vi "ws_users logout user.vi"(6 "Current User":T2, 7 "httpRequestID":u32, 8 "error in (no error)":errorcluster, 10 "Username to Logout (\"\")":string, 11 "Connection Refnum":T1) -> (0 "error out":errorcluster, 3 "Connection Refnum":T1)   [LabVIEW 2011]
uses:
  server/database/Users/User Record.ctl
  SI.LIB/ODBC/SQL Controls/Connection Refnum.ctl
  <vilib>/wsapi/NI_WebServices.lvlib
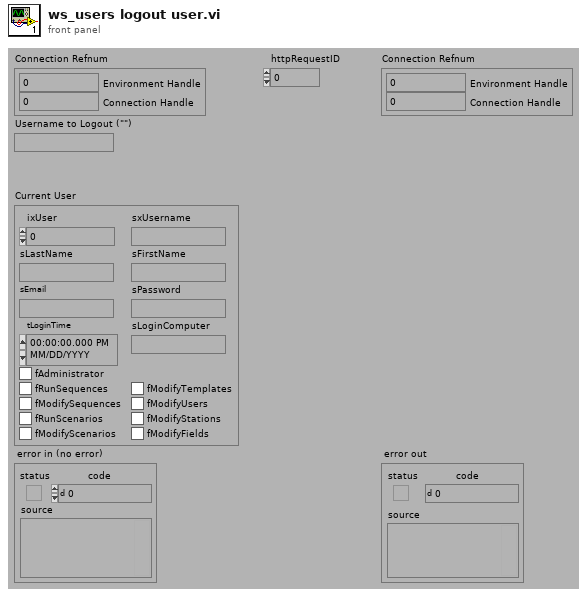
[diagram p1: front panel]
types:
  T1 = typedef "Connection Refnum.ctl" = cluster{"Environment Handle":i32, "Connection Handle":i32}
  T2 = typedef "User Record.ctl" = cluster{"ixUser":i32, "sxUsername":string, "sLastName":string, "sFirstName":string, "sEmail":string, "sPassword":string, "tLoginTime":timestamp, "sLoginComputer":string, "fAdministrator":bool, "fRunSequences":bool, "fModifySequences":bool, "fRunScenarios":bool, "fModifyScenarios":bool, "fModifyTemplates":bool, "fModifyUsers":bool, "fModifyStations":bool, "fModifyFields":bool}
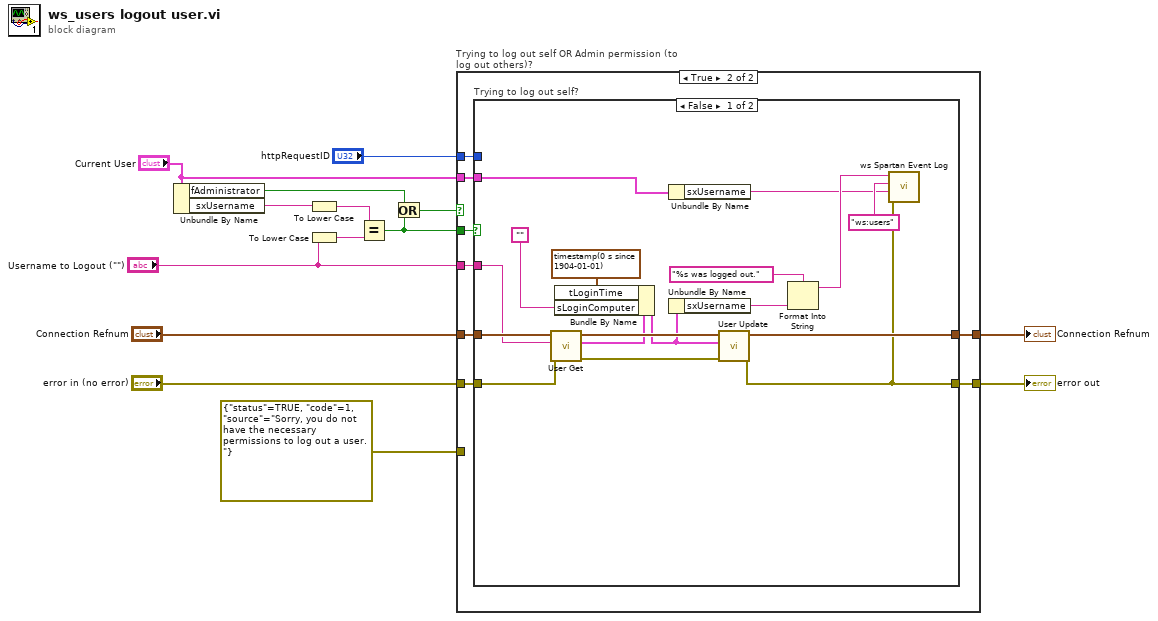
[diagram p0: block diagram]
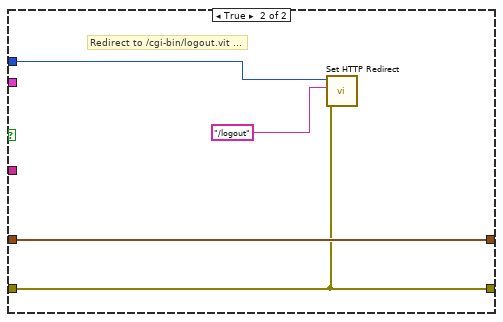
[diagram p3: hidden frame]
diagram:
  n1 = Unbundle By Name("Current User") -> ("fAdministrator"=w6:bool, "sxUsername"=w8:string)
  n2 = To Lower Case(string=w8) -> (all lower case string=w7:string)
  n3 = To Lower Case(string="Username to Logout (\"\")") -> (all lower case string=w9:string)
  n4 = Equal?(x=w7, y=w9) -> (x = y?=w2:bool)
  n5 = Or(x=w6, y=w2) -> (x .or. y?=w5:bool)
  n6 = case "Trying to log out self OR Admin permission (to log out others)?" shown="True" w5 {
    tunnel: "error in (no error)" -> [_ w24]
    tunnel: "Connection Refnum" -> [w16 w23]
    tunnel: [w16 w22] -> w12
    tunnel: [w15 w21] -> w11
    tunnel: "Username to Logout (\"\")" -> [_ w20]
    tunnel: errorcluster {"status"=TRUE, "code"=1, "source"="Sorry, you do not have the necessary permissions to log out a user."} ("error out") -> [w15 _]
    tunnel: "Current User" -> [_ w18]
    tunnel: w2 -> [_ w19]
    tunnel: "httpRequestID" -> [_ w17]
    frame False {
    }
    frame True {
      n7 = case "Trying to log out self?" shown="False" w19 {
        tunnel: w24 -> [w38 w44]
        tunnel: w23 -> [w37 w45]
        tunnel: [w36 w45] -> w22
        tunnel: [w33 w44] -> w21
        tunnel: w20 -> [w34 _]
        tunnel: w18 -> [w27 _]
        tunnel: w17 -> [_ w43]
        frame False {
          n8 = call "User Get.vi"("error in (no error)"=w38, "sxUsername (\"\")"=w34, "Connection Refnum"=w37) -> ("error out"=w40:errorcluster, "User"=w39:T2, "Connection Refnum"=w41:T1)  [unwired: 6 out]
          n9 = Bundle By Name(cluster=w39, "tLoginTime"=timestamp(0 s since 1904-01-01), "sLoginComputer"="") -> (w32:T2)
          n10 = Unbundle By Name(w27) -> ("sxUsername"=w26:string)
          n11 = Unbundle By Name(w32) -> ("sxUsername"=w30:string)
          n12 = call "User Update.vi"("error in (no error)"=w40, "User Record"=w32, "Connection Refnum"=w41) -> ("error out"=w33:errorcluster, "dup Connection Refnum"=w36:T1)  [unwired: 7 out]
          n13 = Format Into String(format string="%s was logged out.", w30) -> (resulting string=w29:string)  [unwired: 2 in, 1 out]
          n14 = call "ws Spartan Event Log.vi"("error in (no error)"=w33, "username (\"\")"=w26, "module (\"\")"="ws:users", "message (\"\")"=w29) -> ()  [unwired: 4 in, 1 out]
        }
        frame True {
          # "Redirect to /cgi-bin/logout.vit ..."
          n15 = call <vilib>:"Set HTTP Redirect.vi"("error in (no error)"=w44, "redirect URL"="/logout" ("New URL (/cgi-bin/testing.vit)"), "httpRequestID"=w43) -> ()  [unwired: 7 in, 2 out]
        }
      }
    }
  }
  "error out" <- w11
  "Connection Refnum" <- w12
